vi "Initialize.vi"(0 "BroadcastRegistry In":T1) -> (4 "BroadcastRegistry Out":T1)   [LabVIEW 2017, in "Communicable State Machine.lvlib"]
doc: "### Initialize.vi\n\n-- <b>Controls</b> --\n- <b>BroadcastRegistry in</b>:\n\n-- <b>Indicators</b> --\n- <b>BroadcastRegistry out</b>:"
uses:
  Communicable State Machine.lvlib
  BroadcastRegistry.ctl
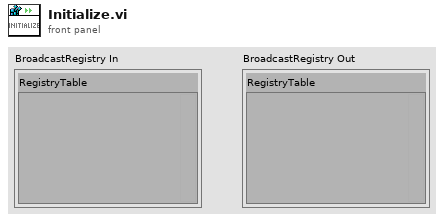
[diagram p1: front panel]
types:
  T1 = typedef "Communicable State Machine.lvlib/BroadcastRegistry.ctl" = cluster{"RegistryTable":variant}
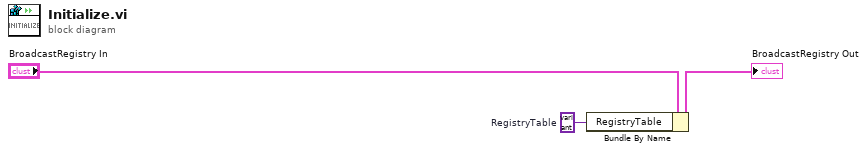
[diagram p0: block diagram]
diagram:
  w1 = variant  # RegistryTable
  n1 = Bundle By Name(cluster="BroadcastRegistry In", "RegistryTable"=w1) -> (→"BroadcastRegistry Out":T1)
